vi "Alerts.vi"(9 "Radiation type":string(combo), 10 "Final voltage":dbl, 11 "Inicial voltage":dbl) -> (0 "Final voltage":dbl, 3 "Stop":bool)   [LabVIEW 2013]
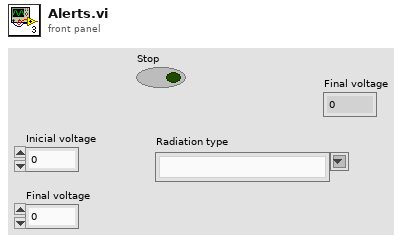
[diagram p1: front panel]
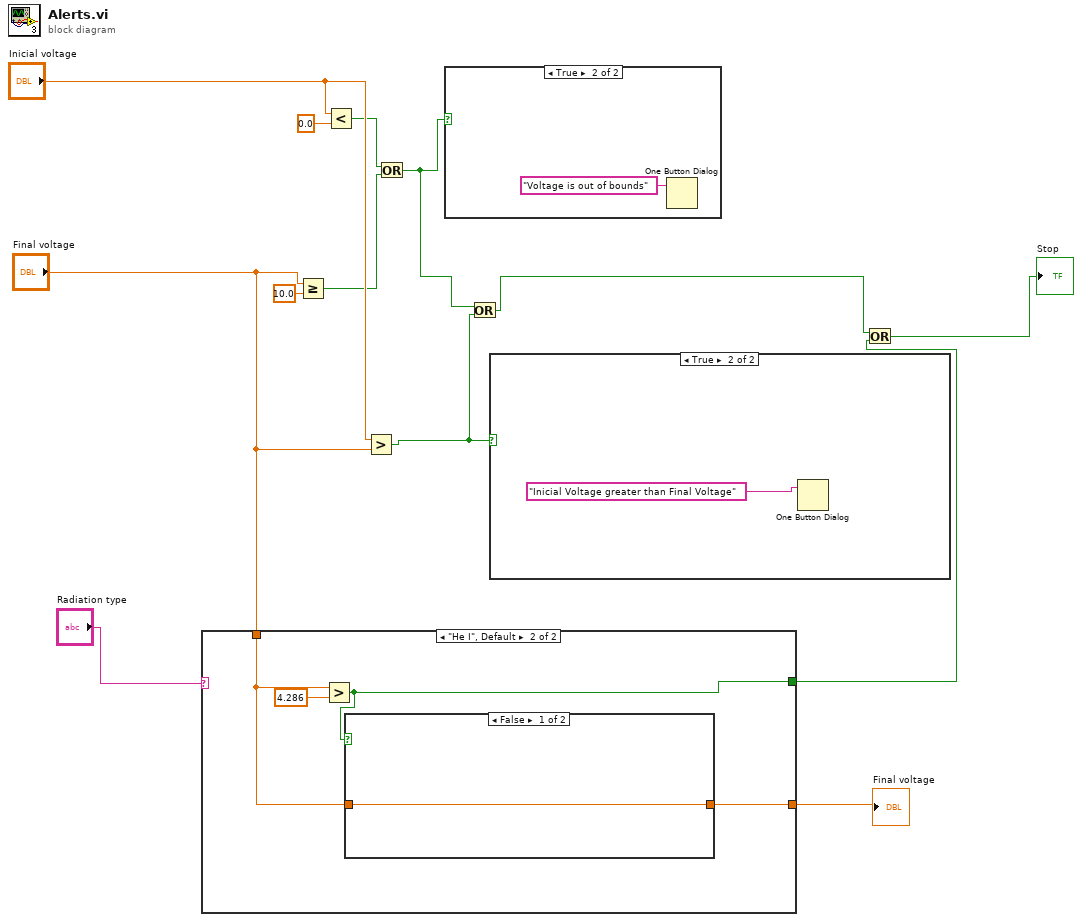
[diagram p0: block diagram]
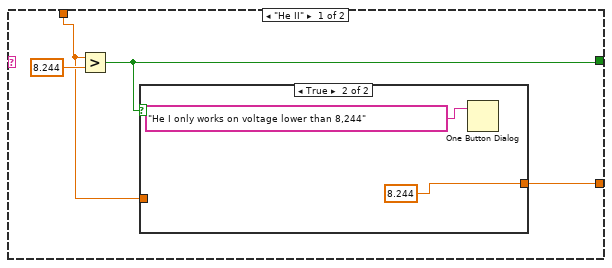
[diagram p2: hidden frame]
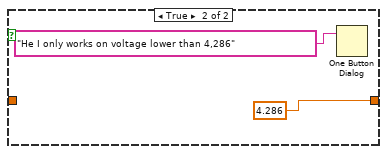
[diagram p4: hidden frame]
diagram:
  n1 = case shown="\"He I\", Default" "Radiation type" {
    tunnel: "Final voltage" -> [w14 w21]
    tunnel: [w17 w23] -> w3
    tunnel: [w15 w22] -> w1
    frame "He II" {
      n2 = Greater?(x=w14, y=8.244) -> (0:w17:bool)
      n3 = case shown="True" w17 {
        tunnel: [w18 8.244 ("Numeric")] -> w15
        tunnel: w14 -> [w18 _]
        frame False {
        }
        frame True {
          n4 = One Button Dialog(message="He I only works on voltage lower than 8,244") -> ()  [unwired: 1 in, 1 out]
        }
      }
    }
    frame "He I", Default {
      n5 = Greater?(x=w21, y=4.286) -> (0:w23:bool)
      n6 = case shown="False" w23 {
        tunnel: [w25 4.286 ("Numeric")] -> w22
        tunnel: w21 -> [w25 _]
        frame False {
        }
        frame True {
          n7 = One Button Dialog(message="He I only works on voltage lower than 4,286") -> ()  [unwired: 1 in, 1 out]
        }
      }
    }
  }
  "Final voltage" <- w1
  n8 = Greater Or Equal?(x="Final voltage", y=10.0) -> (x >= y?=w12:bool)
  n9 = Less?(x="Inicial voltage", y=0.0) -> (x < y?=w11:bool)
  n10 = Greater?(x="Inicial voltage", y="Final voltage") -> (0:w8:bool)
  n11 = Or(x=w11, y=w12) -> (x .or. y?=w7:bool)
  n12 = case shown="True" w7 {
    frame False {
    }
    frame True {
      n13 = One Button Dialog(message="Voltage is out of bounds") -> ()  [unwired: 1 in, 1 out]
    }
  }
  n14 = Or(x=w7, y=w8) -> (x .or. y?=w4:bool)
  n15 = case shown="True" w8 {
    frame False {
    }
    frame True {
      n16 = One Button Dialog(message="Inicial Voltage greater than Final Voltage") -> ()  [unwired: 1 in, 1 out]
    }
  }
  n17 = Or(x=w4, y=w3) -> (x .or. y?=→"Stop":bool)
